vi "Command (read) - IE.vi"(7 "timeout ms (100)":i32=100, 8 "error in (no error)":errorcluster, 10 "IP":string, 11 "connection ID in":refnum<k16>) -> (0 "error out":errorcluster, 2 "Encoder":i32, 3 "connection ID out":refnum<k16>)   [LabVIEW 2016, in "SMD-7615.lvlib" / "eSCL.lvlib"]
doc: "IE - Immediate Encoder\nRequests present encoder position."
uses:
  eSCL.lvlib
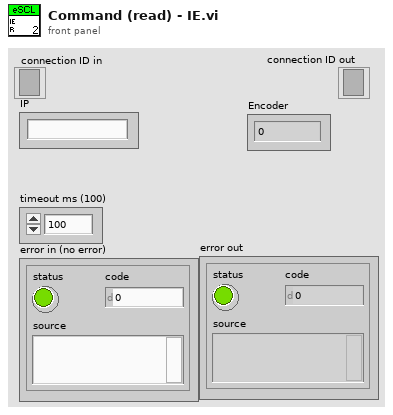
[diagram p1: front panel]
types:
  T1 = typedef "SMD-7615.lvlib/eSCL.lvlib/UDP Received Data.ctl" = cluster{"Received String":string, "eSCL Cmd":string, "Data":string}
  T2 = cluster{"Received String":i32, "eSCL Cmd":i32, "Data":i32}
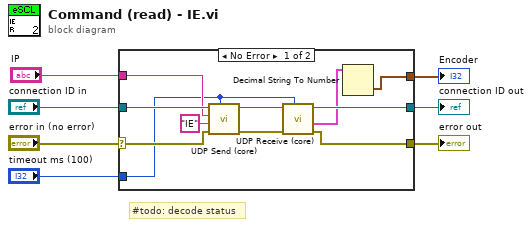
[diagram p0: block diagram]
diagram:
  # "#todo: decode status"
  n1 = case shown="No Error" "error in (no error)" {
    selector: "error in (no error)" -> [w14 w19]
    tunnel: "connection ID in" -> [w13 w20]
    tunnel: [w16 w20] -> w5
    tunnel: [w15 w19] -> w4
    tunnel: "IP" -> [w12 _]
    tunnel: "timeout ms (100)" -> [w10 _]
    tunnel: [w8 _] -> w1
    frame No Error {
      n2 = call "UDP Send (core).vi"("timeout ms (100)"=w10, "error in (no error)"=w14, "Data"="IE", "IP"=w12, "connection ID in"=w13) -> ("error out"=w18:errorcluster, "connection ID out"=w17:refnum<k16>)  [unwired: 5 in]
      n3 = call "UDP Receive (core).vi"("timeout ms (100)"=w10, "error in (no error)"=w18, "connection ID in"=w17) -> ("error out"=w15:errorcluster, "Received Data"=w9:T1, "connection ID out"=w16:refnum<k16>)  [unwired: 5 in, 1 out]
      n4 = Decimal String To Number(string=w9) -> (number=w8:T2)  [unwired: 2 in, 1 out]
    }
    frame Error {
    }
  }
  "connection ID out" <- w5
  "error out" <- w4
  "Encoder" <- w1
